vi "Main.vi"() -> ()   [LabVIEW 2018]
panel:
  out "Arduino distance [mm]":dbl
  out "retransmission count":dbl
  out "PLC distance [mm]":dbl
  out "elapsed time [s]":dbl
  in  "Stop":bool
  in  "Motor relative position":dbl(knob) scale=0.0..1999.0
  out "Calibration Curve":cluster{"X":dbl, "Y":dbl}[](graph)
  in  "baud rate (38400)":u32=9600
  in  "VISA resource name":refnum<visa-resource-name>
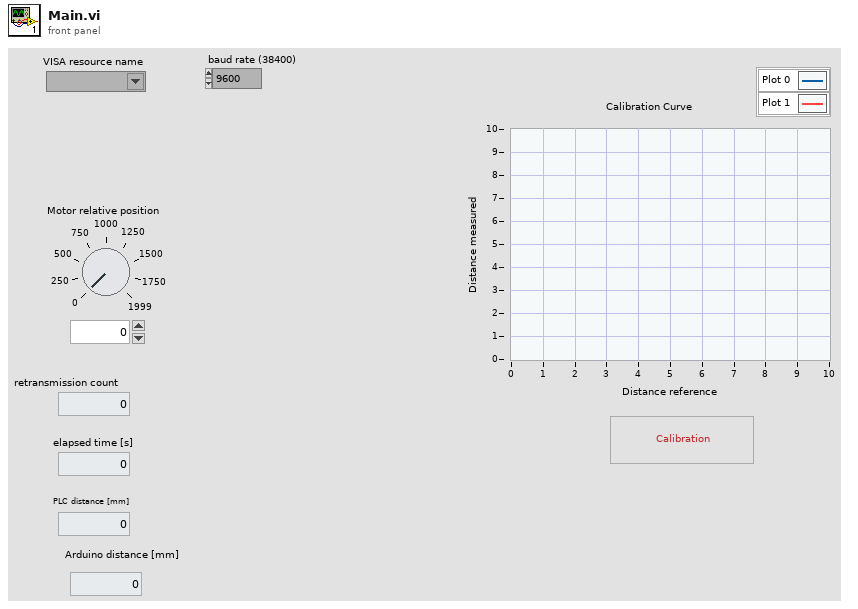
[diagram p1: front panel]
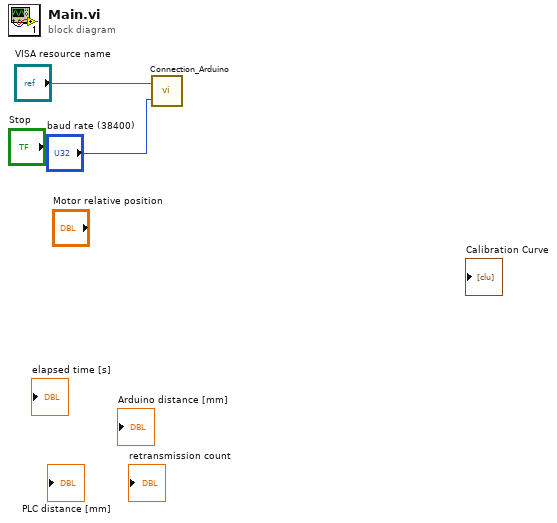
[diagram p0: block diagram]
diagram:
  n1 = call "Connection_Arduino.vi"("baud rate (9600)"="baud rate (38400)", "VISA resource name"="VISA resource name") -> ()  [unwired: 2 out]
